vi "libtiff3_writeScanLine_contig_RGB.vi"(7 "totalpages":i32, 8 "error in (no error)":errorcluster, 9 "page":u32, 10 "Data":i16[][][](array[numeric]), 11 "Handle":i32) -> (0 "error out":errorcluster, 3 "Handle out":i32)   [LabVIEW 2012]
doc: "Write a RGB page (contig. color planes) using LIBTIFFwriteScanLine to a file previously open for writing"
uses:
  C:/Program Files (x86)/GnuWin32/bin/libtiff3.dll
panel:
  out "status_compression":i32
  out "status width":i32
  out "status_length":i32
  out "status_spp":i32
  out "status_bps":i32
  out "status_orientation":i32
  out "status_planarconfig":i32
  out "status_photo":i32
  out "status_writscanline":i32
  out "status_subfile":i32
  out "status_writedir":i32
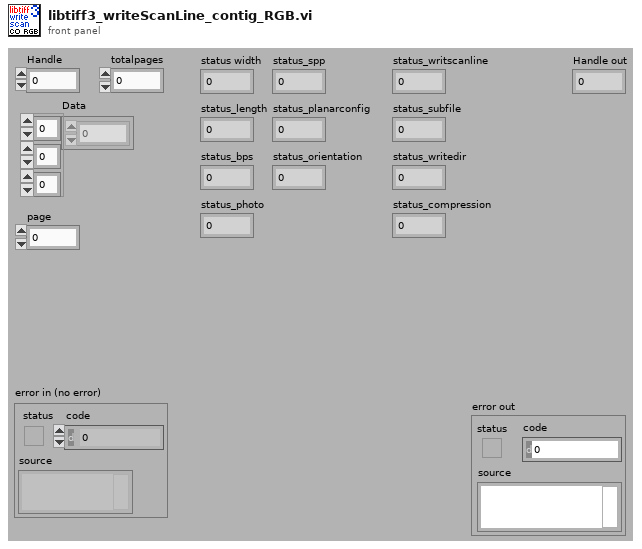
[diagram p1: front panel]
types:
  T1 = enum16{"Vertical flip", "Horizontal flip", "transpose", "rotate 90", "rotate 180", "rotate 270", "Diagonal flip"}
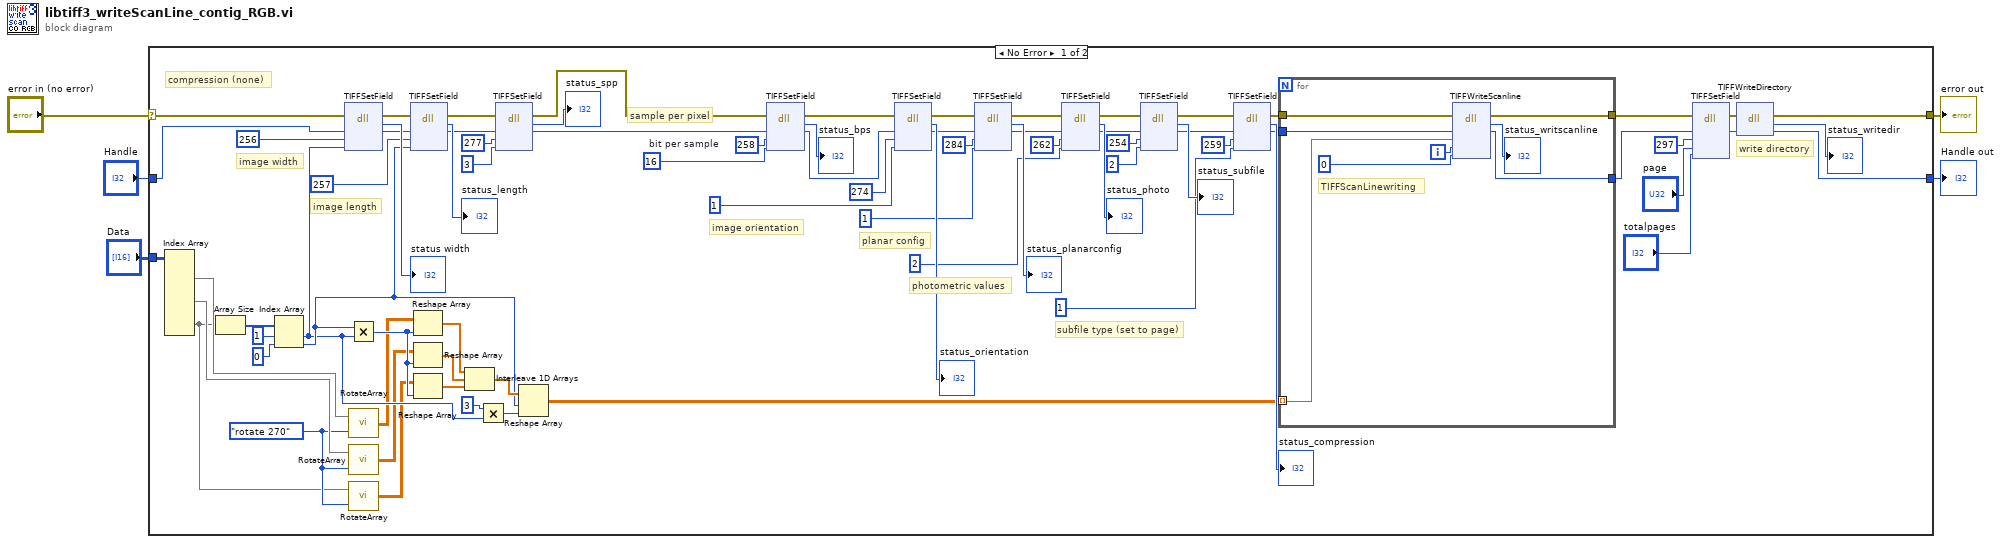
[diagram p0: block diagram]
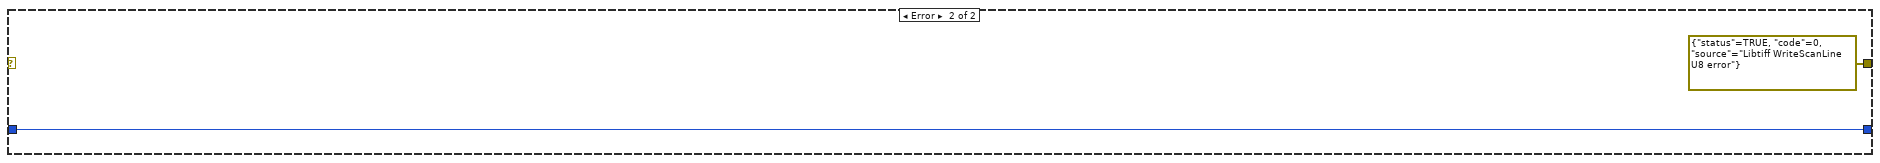
[diagram p2: hidden frame]
diagram:
  n1 = case shown="No Error" "error in (no error)" {
    selector: "error in (no error)" -> [w79 _]
    tunnel: "Handle" -> [w78 w91]
    tunnel: [w81 w91] -> w4
    tunnel: [w80 errorcluster {"status"=TRUE, "code"=0, "source"="Libtiff WriteScanLine U8 error"} ("error out")] -> w3
    tunnel: "Data" -> [w12 _]
    frame No Error {
      w9 = T1."rotate 270" ("Method")
      w33 = u32 16  # bit per sample
      # "compression (none)"
      # "write directory"
      # "subfile type (set to page)"
      # "photometric values"
      # "planar config"
      # "image orientation"
      # "sample per pixel"
      # "image length"
      # "image width"
      n2 = Index Array(array=w12) -> (element #1=w11:i16[][], element #2=w10:i16[][], element #3=w6:i16[][])  [unwired: 9 in]
      n3 = Array Size(array=w6) -> (size(s)=w46:i32[])
      n4 = Index Array(array=w46, index #1=1 ("index"), index #2=0 ("index")) -> (element #1=w14:i32, element #2=w15:i32)
      n5 = dll-call lib="C:/Program Files (x86)/GnuWin32/bin/libtiff3.dll" fn="TIFFSetField"(error in=w79, "Handle"=w78, "TIFF_tag"=256, "Value"=w14) -> (error out=w41:errorcluster, →"status width":i32, "Handle"=w75:i32)  [unwired: 4 in, 1 out]
      n6 = Multiply(x=w15, y=w14) -> (x*y=w23:i32)
      n7 = call "RotateArray.vi"("Method"=w9, "Input"=w11) -> ("Output"=w13:dbl[][])
      n8 = call "RotateArray.vi"("Method"=w9, "Input"=w10) -> ("Output"=w8:dbl[][])
      n9 = call "RotateArray.vi"("Method"=w9, "Input"=w6) -> ("Output"=w7:dbl[][])
      n10 = dll-call lib="C:/Program Files (x86)/GnuWin32/bin/libtiff3.dll" fn="TIFFSetField"(error in=w41, "Handle"=w75, "TIFF_tag"=257, "value"=w15) -> (error out=w40:errorcluster, →"status_length":i32, "Handle"=w72:i32)  [unwired: 4 in, 1 out]
      n11 = Reshape Array(w13, w23) -> (w22:dbl[])
      n12 = Reshape Array(w8, w23) -> (w21:dbl[])
      n13 = Reshape Array(w7, w23) -> (w20:dbl[])
      n14 = Interleave 1D Arrays(w22, w21, w20) -> (w19:dbl[])
      n15 = Multiply(x=3, y=w14) -> (x*y=w16:i32)
      n16 = dll-call lib="C:/Program Files (x86)/GnuWin32/bin/libtiff3.dll" fn="TIFFSetField"(error in=w40, "Handle"=w72, "TIFF_tag"=277, "value"=u32 3) -> (error out=w39:errorcluster, →"status_spp":i32, "Handle"=w69:i32)  [unwired: 4 in, 1 out]
      n17 = Reshape Array(w19, w15, w16) -> (w17:dbl[][])
      n18 = dll-call lib="C:/Program Files (x86)/GnuWin32/bin/libtiff3.dll" fn="TIFFSetField"(error in=w39, "Handle"=w69, "TIFF_tag"=258, "value"=w33) -> (error out=w38:errorcluster, →"status_bps":i32, "Handle"=w66:i32)  [unwired: 4 in, 1 out]
      n19 = dll-call lib="C:/Program Files (x86)/GnuWin32/bin/libtiff3.dll" fn="TIFFSetField"(error in=w38, "Handle"=w66, "TIFF_tag"=274, "value"=u32 1) -> (error out=w37:errorcluster, →"status_orientation":i32, "Handle"=w62:i32)  [unwired: 4 in, 1 out]
      n20 = dll-call lib="C:/Program Files (x86)/GnuWin32/bin/libtiff3.dll" fn="TIFFSetField"(error in=w37, "Handle"=w62, "TIFF_tag"=284, "value"=u32 1) -> (error out=w36:errorcluster, →"status_planarconfig":i32, "Handle"=w58:i32)  [unwired: 4 in, 1 out]
      n21 = dll-call lib="C:/Program Files (x86)/GnuWin32/bin/libtiff3.dll" fn="TIFFSetField"(error in=w36, "Handle"=w58, "TIFF_tag"=262, "value"=u32 2) -> (error out=w35:errorcluster, →"status_photo":i32, "Handle"=w53:i32)  [unwired: 4 in, 1 out]
      n22 = dll-call lib="C:/Program Files (x86)/GnuWin32/bin/libtiff3.dll" fn="TIFFSetField"(error in=w35, "Handle"=w53, "TIFF_tag"=254, "value"=u32 2) -> (error out=w34:errorcluster, →"status_subfile":i32, "Handle"=w43:i32)  [unwired: 4 in, 1 out]
      n23 = dll-call lib="C:/Program Files (x86)/GnuWin32/bin/libtiff3.dll" fn="TIFFSetField"(error in=w34, "Handle"=w43, "TIFF_tag"=259, "value"=u32 1) -> (error out=w25:errorcluster, →"status_compression":i32, "Handle"=w26:i32)  [unwired: 4 in, 1 out]
      n24 = for {
        tunnel: [w88] -> w31
        tunnel: [w82] -> w24
        tunnel: w26 -> [w86]
        tunnel: w25 -> [w87]
        tunnel: w17 -> [w83] mode=indexing
        i -> [w85]
        # "TIFFScanLinewriting"
        n25 = dll-call lib="C:/Program Files (x86)/GnuWin32/bin/libtiff3.dll" fn="TIFFWriteScanline"(error in=w87, "Handle"=w86, "buffer"=w83, "row"=w85, "sample"=0) -> (error out=w82:errorcluster, "return type"=→"status_writscanline":i32, "Handle"=w88:i32)  [unwired: 5 in, 1 out]
      }
      n26 = dll-call lib="C:/Program Files (x86)/GnuWin32/bin/libtiff3.dll" fn="TIFFSetField"(error in=w24, "Handle"=w31, "TIFF_tag"=297, "page"="page", "totalpages"="totalpages") -> (error out=w28:errorcluster, "Handle"=w27:i32)  [unwired: 5 in, 2 out]
      n27 = dll-call lib="C:/Program Files (x86)/GnuWin32/bin/libtiff3.dll" fn="TIFFWriteDirectory"(error in=w28, "Handle"=w27) -> (error out=w80:errorcluster, →"status_writedir":i32, "Handle"=w81:i32)  [unwired: 2 in, 1 out]
    }
    frame Error {
    }
  }
  "Handle out" <- w4
  "error out" <- w3
